vi "4155C Config Sampling Measurements FPP v3.0.vi"(0 "VISA session":refnum<visa-resource-name>, 1 "Gate Compliance":dbl format="%.2f", 2 "FPP - Source":u32(ring)=6 items=["SMU1  ", "SMU2  ", "SMU3  ", "SMU4  ", "SMU5  ", "SMU6  ", "VSU1  ", "VSU2  "], 3 "FPP - Drain":u32(ring)=1 items=["SMU1  ", "SMU2  ", "SMU3  ", "SMU4  ", "SMU5  ", "SMU6  ", "VSU1  ", "VSU2  "], 4 "Drain Compliance":dbl format="%.2f", 5 "error in (no error)":errorcluster, 6 "Num Points":i16=1 min=1 max=1001, 7 "Timings":T2={"integration time"=0, "Short/Long integration time"=0.00064, "hold time (sec)"=0.0, "delay time (sec)"=0.0, "Step Time (0 disables)"=0.0, "sweep method"=0, "Pulse period"=0.005, "Base voltage"=0.0, "Pulse width"=0.0005} {"Pulse width" min=0.0005 max=0.1 step=0.0001 format="%.4f"; "Base voltage" min=-100.0 max=100.0 format="%^.4e"; "Pulse period" min=0.005 max=1.0 step=0.0001 format="%.4f"; "sweep method" items=["Continuous", "Pulsed"]; "Step Time (0 disables)" format="%.2f"; "delay time (sec)" min=0.0 format="%.4f"; "hold time (sec)" min=0.0 format="%.4f"; "Short/Long integration time" min=0.0 format="%^.0e"; "integration time" scale=0.0..2.0}, 8 "FPP - Gate":u32(ring)=2 items=["SMU1  ", "SMU2  ", "SMU3  ", "SMU4  ", "SMU5  ", "SMU6  ", "VSU1  ", "VSU2  "], 9 "FPP - Probe 1":u32(ring) items=["SMU1  ", "SMU2  ", "SMU3  ", "SMU4  ", "SMU5  ", "SMU6  ", "VSU1  ", "VSU2  "], 10 "Vg":dbl min=-100.0 max=100.0 format="%.2f", 11 "Vd":dbl min=-100.0 max=100.0 format="%.2f", 12 "Display on/off":bool, 13 "Sample time":dbl min=0.0 max=100000000000.0 format="%.2f", 15 "Sampling mode":u32(slide) scale=0.0..4.0, 16 "FPP - Probe 2":u32(ring)=3 items=["SMU1  ", "SMU2  ", "SMU3  ", "SMU4  ", "SMU5  ", "SMU6  ", "VSU1  ", "VSU2  "], 18 "Standby":T1) -> (14 "dup VISA resource name":refnum<visa-resource-name>, 19 "error out":errorcluster)   [LabVIEW 2016]
doc: "This VI configures the primary sweep source (VAR1) for a sweep mode measurement. \n* This VI does not perform error checking on MEASUREMENT MODE or UNIT TYPE of VAR1, therefore it is the application programmer's responsibility to make certain this VI is used in the proper mode."
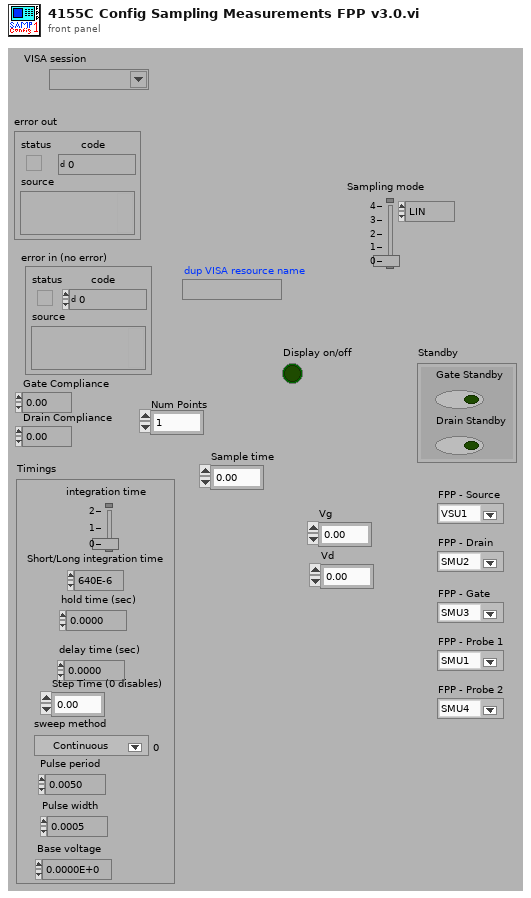
[diagram p1: front panel]
types:
  T1 = cluster{"Gate Standby":bool, "Drain Standby":bool}
  T2 = cluster{"integration time":u32, "Short/Long integration time":dbl, "hold time (sec)":dbl, "delay time (sec)":dbl, "Step Time (0 disables)":dbl, "sweep method":u16, "Pulse period":dbl, "Base voltage":dbl, "Pulse width":dbl}
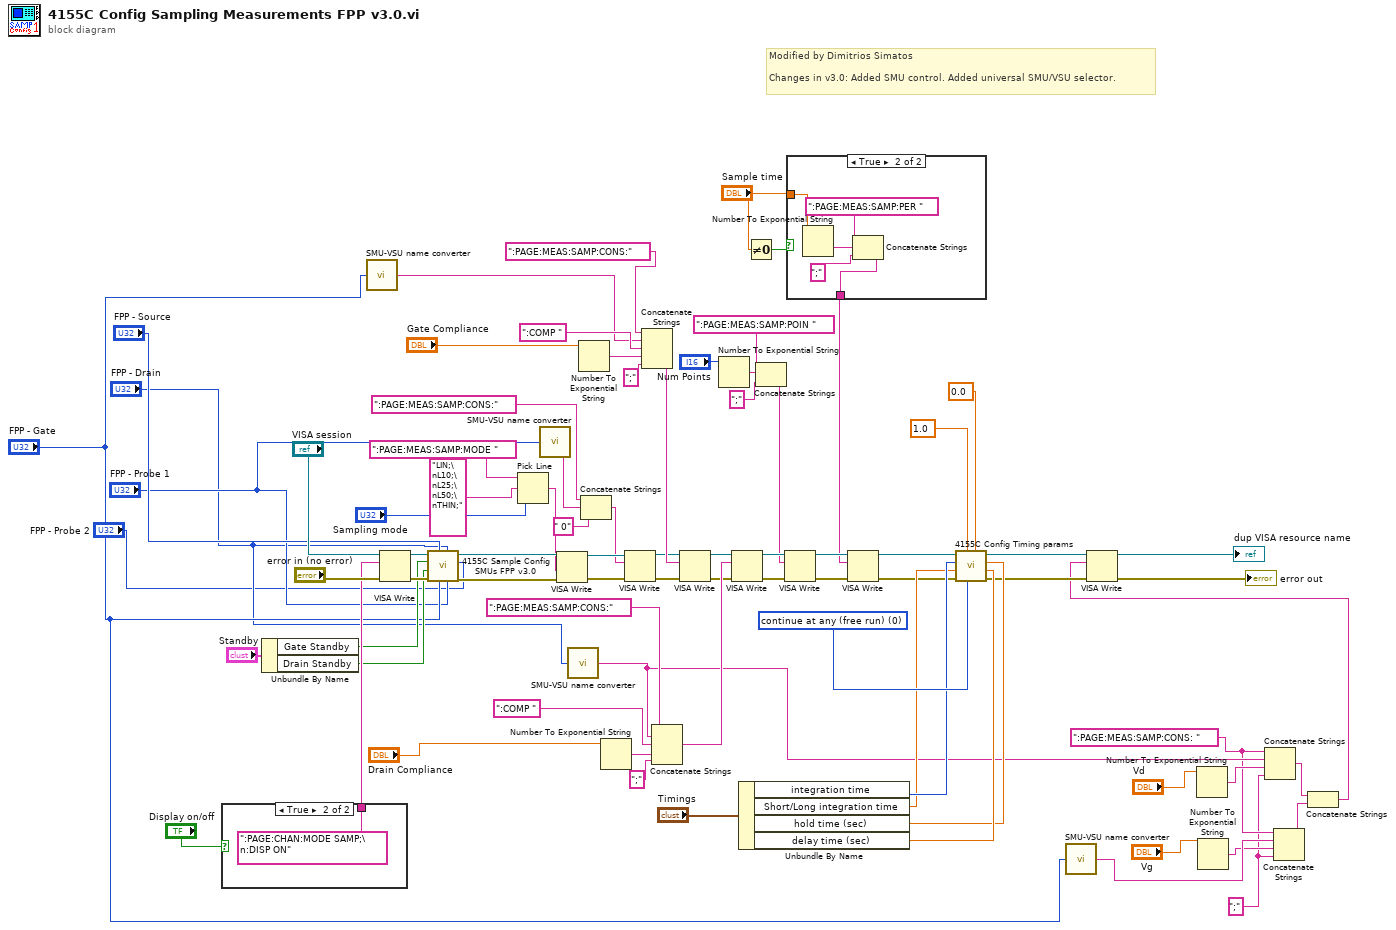
[diagram p0: block diagram]
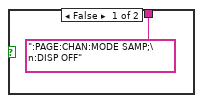
[diagram p2: hidden frame]
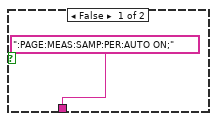
[diagram p3: hidden frame]
diagram:
  w4 = ";" ("Substring")
  w7 = ":PAGE:MEAS:SAMP:CONS: " ("write buffer (\"\")")
  w66 = u8 0 items=["continue at any (free run)", "stop at any abnorm", "stop at compliance"] ("stop condition (free run:0)")
  # "Modified by Dimitrios Simatos\n\nChanges in v3.0: Added SMU control. Added universal SMU/VSU selector."
  n1 = case shown="True" "Display on/off" {
    tunnel: [":PAGE:CHAN:MODE SAMP;\n:DISP OFF" ("write buffer (\"\")") ":PAGE:CHAN:MODE SAMP;\n:DISP ON" ("write buffer (\"\")")] -> w39
    frame False {
    }
    frame True {
    }
  }
  n2 = Unbundle By Name("Standby") -> ("Gate Standby"=w29:bool, "Drain Standby"=w28:bool)
  n3 = call "SMU-VSU name converter.vi"("unit to configure"="FPP - Gate") -> ("SMU/VSU to be configured"=w19:string)
  n4 = VISA Write(VISA resource name="VISA session", write buffer=w39, error in (no error)="error in (no error)") -> (VISA resource name out=w57:refnum<visa-resource-name>, error out=w56:errorcluster)  [unwired: 1 out]
  n5 = call "4155C Sample Config SMUs FPP v3.0.vi"("FPP - Probe 2"="FPP - Probe 2", "FPP - Probe 1"="FPP - Probe 1", "FPP - Drain"="FPP - Drain", "FPP - Gate"="FPP - Gate", "FPP - Source"="FPP - Source", "error in (no error)"=w56, "Drain Standby"=w28, "Gate Standby"=w29, "VISA resource name in"=w57) -> ("error out"=w36:errorcluster, "VISA Resource Name out"=w35:refnum<visa-resource-name>)  [unwired: 1 in]
  n6 = Pick Line(string ("")=":PAGE:MEAS:SAMP:MODE ", multi-line string="LIN;\nL10;\nL25;\nL50;\nTHIN;", line index="Sampling mode") -> (output string=w31:string)
  n7 = call "SMU-VSU name converter.vi"("unit to configure"="FPP - Probe 1") -> ("SMU/VSU to be configured"=w16:string)
  n8 = VISA Write(VISA resource name=w35, write buffer=w31, error in (no error)=w36) -> (VISA resource name out=w38:refnum<visa-resource-name>, error out=w37:errorcluster)  [unwired: 1 out]
  n9 = call "SMU-VSU name converter.vi"("unit to configure"="FPP - Drain") -> ("SMU/VSU to be configured"=w13:string)
  n10 = Number To Exponential String(number="Gate Compliance") -> (E-format string=w73:string)  [unwired: 3 in]
  n11 = Concatenate Strings(":PAGE:MEAS:SAMP:CONS:" ("write buffer (\"\")"), w16, " 0" ("write buffer (\"\")")) -> (w18:string)
  n12 = Number To Exponential String(number="Drain Compliance") -> (E-format string=w75:string)  [unwired: 3 in]
  n13 = VISA Write(VISA resource name=w38, write buffer=w18, error in (no error)=w37) -> (VISA resource name out=w71:refnum<visa-resource-name>, error out=w70:errorcluster)  [unwired: 1 out]
  n14 = Concatenate Strings(":PAGE:MEAS:SAMP:CONS:", w19, ":COMP ", w73, ";" ("Substring")) -> (w74:string)
  n15 = Concatenate Strings(":PAGE:MEAS:SAMP:CONS:", w13, ":COMP ", w75, ";" ("Substring")) -> (w78:string)
  n16 = VISA Write(VISA resource name=w71, write buffer=w74, error in (no error)=w70) -> (VISA resource name out=w69:refnum<visa-resource-name>, error out=w68:errorcluster)  [unwired: 1 out]
  n17 = Number To Exponential String(number="Num Points") -> (E-format string=w54:string)  [unwired: 3 in]
  n18 = VISA Write(VISA resource name=w69, write buffer=w78, error in (no error)=w68) -> (VISA resource name out=w79:refnum<visa-resource-name>, error out=w80:errorcluster)  [unwired: 1 out]
  n19 = Unbundle By Name("Timings") -> ("integration time"=w63:u32, "Short/Long integration time"=w60:dbl, "hold time (sec)"=w64:dbl, "delay time (sec)"=w65:dbl)
  n20 = Not Equal To 0?(x="Sample time") -> (x != 0?=w46:bool)
  n21 = Concatenate Strings(":PAGE:MEAS:SAMP:POIN " ("write buffer (\"\")"), w54, ";" ("Substring")) -> (w48:string)
  n22 = VISA Write(VISA resource name=w79, write buffer=w48, error in (no error)=w80) -> (VISA resource name out=w45:refnum<visa-resource-name>, error out=w44:errorcluster)  [unwired: 1 out]
  n23 = case shown="True" w46 {
    tunnel: "Sample time" -> [_ w87]
    tunnel: [":PAGE:MEAS:SAMP:PER:AUTO ON;" w84] -> w41
    frame False {
    }
    frame True {
      n24 = Number To Exponential String(number=w87) -> (E-format string=w88:string)  [unwired: 3 in]
      n25 = Concatenate Strings(":PAGE:MEAS:SAMP:PER " ("Substring"), w88, ";" ("Substring")) -> (w84:string)
    }
  }
  n26 = VISA Write(VISA resource name=w45, write buffer=w41, error in (no error)=w44) -> (VISA resource name out=w42:refnum<visa-resource-name>, error out=w43:errorcluster)  [unwired: 1 out]
  n27 = call "4155C Config Timing params.vi"("delay time (sec)"=w65, "hold time (sec)"=w64, "Step Time (0 disables)"=0.0, "stop condition (free run:0)"=w66, "wait time parameter"=1.0, "error in (no error)"=w43, "Short/Long integration time"=w60, "integration time"=w63, "VISA session"=w42) -> ("error out"=w23:errorcluster, "dup VISA resource name"=w24:refnum<visa-resource-name>)  [unwired: 1 in]
  n28 = call "SMU-VSU name converter.vi"("unit to configure"="FPP - Gate") -> ("SMU/VSU to be configured"=w6:string)
  n29 = Number To Exponential String(number="Vd") -> (E-format string=w26:string)  [unwired: 3 in]
  n30 = Number To Exponential String(number="Vg") -> (E-format string=w5:string)  [unwired: 3 in]
  n31 = Concatenate Strings(w7, w13, w26, w4) -> (w3:string)
  n32 = Concatenate Strings(w7, w6, w5, w4) -> (w2:string)
  n33 = Concatenate Strings(w3, w2) -> (w1:string)
  n34 = VISA Write(VISA resource name=w24, write buffer=w1, error in (no error)=w23) -> (VISA resource name out=→"dup VISA resource name":refnum<visa-resource-name>, error out=→"error out":errorcluster)  [unwired: 1 out]
